vi "Derivative.vi"   [LabVIEW 2016, in "xy_utilities.lvlib"]
uses:
  xy_utilities.lvlib
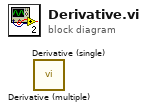
[diagram p0: block diagram]
diagram:
  n1 = call "Derivative (multiple).vi"() -> ()  [unwired: 10 in, 2 out]
  n2 = call "Derivative (single).vi"() -> ()  [unwired: 10 in, 2 out]
